vi "Ready for next Waveform package.vi"(9 "DRAM pack index in":T1, 10 "DRAM pack index out":T1, 11 "output valid?":bool) -> (3 "Ready for next package":bool)   [LabVIEW 2015]
uses:
  DRAM data index.ctl
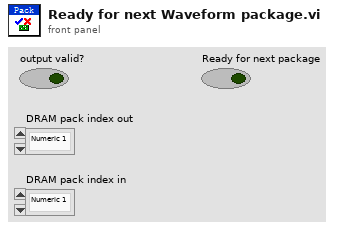
[diagram p1: front panel]
types:
  T1 = typedef "DRAM data index.ctl" = enum16{"Numeric 1", "Numeric 2", "Numeric 3", "Numeric 4", "Numeric 5", "Numeric 6", "Numeric 7", "Numeric 8", "Numeric 9", "Numeric 10", "Numeric 11", "Numeric 12", "Numeric 13", "Numeric 14", "Numeric 15", "Numeric 16"}
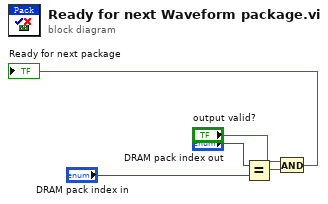
[diagram p0: block diagram]
diagram:
  n1 = Equal?(x="DRAM pack index out", y="DRAM pack index in") -> (x = y?=w3:bool)
  n2 = And(x="output valid?", y=w3) -> (x .and. y?=→"Ready for next package":bool)
